vi "SubVI_CaseSelectorLR_auto.vi"() -> ()   [LabVIEW 2017]
panel:
  out "Left":bool
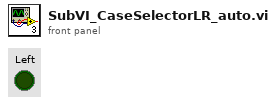
[diagram p1: front panel]
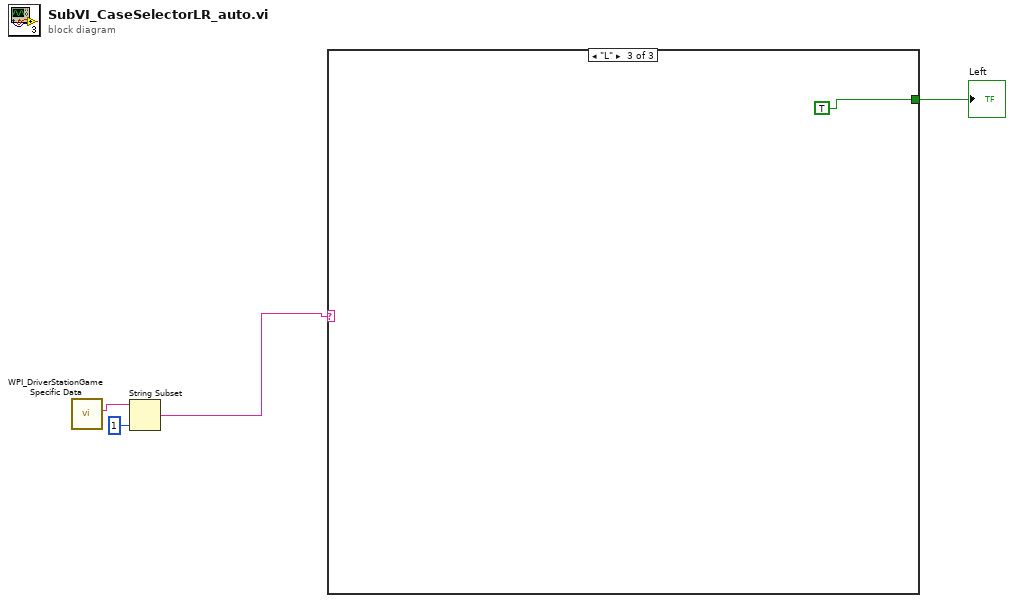
[diagram p0: block diagram]
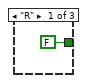
[diagram p2: hidden frame]
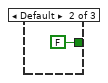
[diagram p3: hidden frame]
diagram:
  n1 = call <vilib>:"WPI_DriverStationGame Specific Data.vi"() -> ("Game Specific Data"=w4:string)  [unwired: 11 in]
  n2 = String Subset(string=w4, length (rest)=1 ("length (rest)")) -> (substring=w2:string)  [unwired: 1 in]
  n3 = case shown="\"L\"" w2 {
    tunnel: [FALSE ("Left") FALSE ("Left") TRUE ("Left")] -> w1
    frame "R" {
    }
    frame Default {
    }
    frame "L" {
    }
  }
  "Left" <- w1
